vi "IMAQ Vision Example folder.vi"() -> (3 "Example Image Path":path)   [LabVIEW 2014]
uses:
  <vilib>/registry/registry.llb/Registry SAM.ctl
  <vilib>/registry/registry.llb/Read Registry Value Simple STR.vi
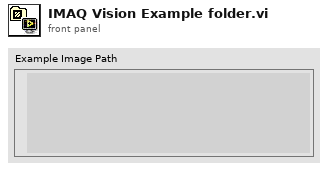
[diagram p1: front panel]
types:
  T1 = typedef "Registry SAM.ctl" = enum32{"KEY_QUERY_VALUE", "KEY_SET_VALUE", "KEY_CREATE_SUB_KEY", "KEY_ENUMERATE_SUB_KEYS", "KEY_NOTIFY", "KEY_CREATE_LINK", "KEY_READ", "KEY_WRITE", "KEY_ALL_ACCESS", "KEY_READ | KEY_WRITE"}
  T2 = typedef "Registry refnum.ctl" = refnum<k1>
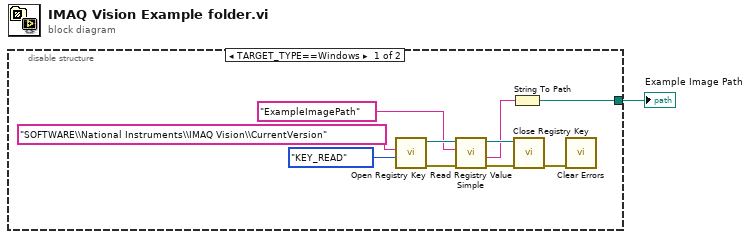
[diagram p0: block diagram]
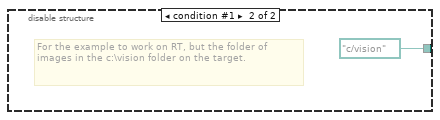
[diagram p2: hidden frame]
diagram:
  n1 = disable-structure shown="TARGET_TYPE==Windows" {
    disable-tunnel: [w3 path "c:/vision"] -> w1
    frame condition #0 (active) {
      n2 = call <vilib>:"Open Registry Key.vi"("security access mask (KEY_READ | KEY_WRITE)"=Registry_SAM."KEY_READ", "subkey"="SOFTWARE\\National Instruments\\IMAQ Vision\\CurrentVersion") -> ("error out"=w10:errorcluster, "refnum out"=w9:T2)  [unwired: 8 in]
      n3 = call-poly <vilib>:"Read Registry Value Simple.vi"("error in (no error)"=w10, "value"="ExampleImagePath", "refnum"=w9) -> ("error out"=w7:errorcluster, "String/Binary data"=w5:string, "refnum out"=w6:T2)  [unwired: 3 in, 1 out]
      n4 = String To Path(string=w5) -> (path=w3:path)
      n5 = call <vilib>:"Close Registry Key.vi"("error in (no error)"=w7, "refnum"=w6) -> ("error out"=w4:errorcluster)  [unwired: 5 in]
      n6 = call <vilib>:"Clear Errors.vi"("error in (no error)"=w4) -> ()  [unwired: 5 in, 2 out]
    }
    frame condition #1 {
      # "For the example to work on RT, but the folder of images in the c:\\vision folder on the target."
    }
  }
  "Example Image Path" <- w1
